vi "Motion@General MotorName Only__Parameter.vi"(1 "ParamterIn":string) -> (0 "ParamterOut":string)   [LabVIEW 2019]
panel:
  in  "Delay":string(combo)
  in  "MotorSelect":string(combo)
  in  "Confirm":bool
  # "Motor@Stop/GetPos/GetState $Motor"
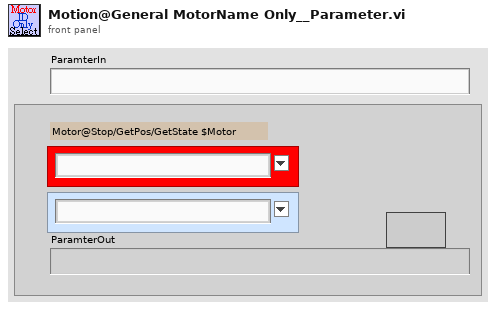
[diagram p1: front panel]
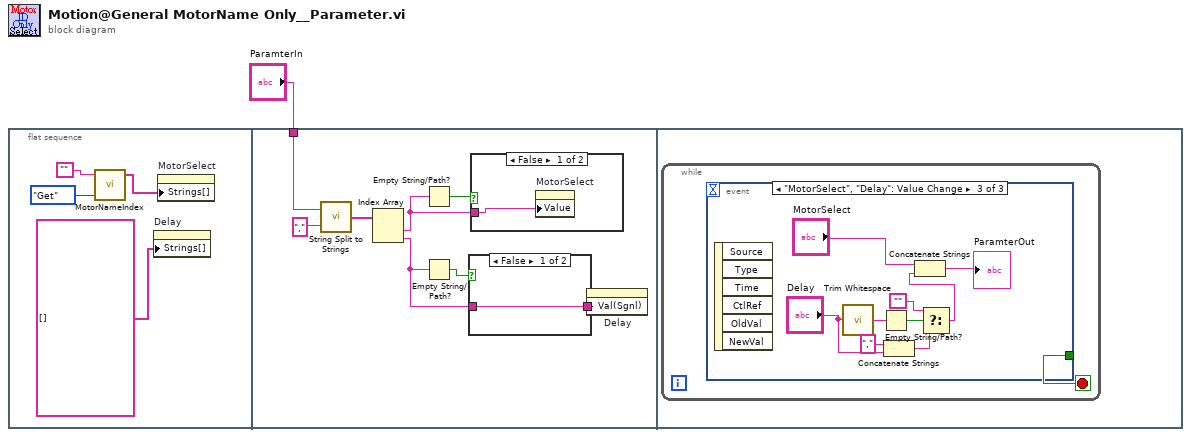
[diagram p0: block diagram]
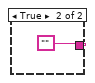
[diagram p2: hidden frame]
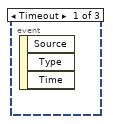
[diagram p4: hidden frame]
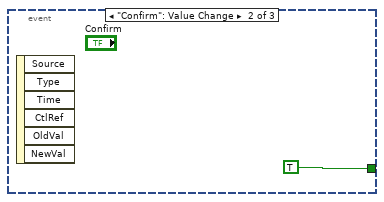
[diagram p5: hidden frame]
diagram:
  n1 = flat-sequence {
    tunnel: "ParamterIn" -> [w11]
    frame #0 {
      n2 = call "MotorNameIndex.vi"("OP"=enum16{"Get", "Update", "Init"}."Get", "MotorName"="") -> ("MotorList"=w2:string[])  [unwired: 1 in, 2 out]
      n3 = property on="Delay" class="CmbBox"("Strings[]"=string[] [] ("Strings []")) -> ()  [unwired: 2 in, 2 out]
      n4 = property on="MotorSelect" class="CmbBox"("Strings[]"=w2) -> ()  [unwired: 2 in, 2 out]
    }
    frame #1 {
      n5 = call "String Split to Strings.vi"("search string/char (-)"=",", "String"=w11) -> ("Array"=w13:string[])
      n6 = Index Array(array=w13) -> (element #1=w9:string, element #2=w6:string)  [unwired: 2 in]
      n7 = Empty String/Path?(string/path=w9) -> (empty?=w10:bool)
      n8 = Empty String/Path?(string/path=w6) -> (empty?=w8:bool)
      n9 = case shown="False" w8 {
        tunnel: [w14 ""] -> w7
        tunnel: w6 -> [w14 _]
        frame False {
        }
        frame True {
        }
      }
      n10 = case shown="False" w10 {
        tunnel: w9 -> [w16 _]
        frame False {
          n11 = property on="MotorSelect" class="CmbBox"("Value"=w16) -> ()  [unwired: 2 in, 2 out]
        }
        frame True {
        }
      }
      n12 = property on="Delay" class="CmbBox"("Val(Sgnl)"=w7) -> ()  [unwired: 2 in, 2 out]
    }
    frame #2 {
      n13 = while {
        stop <- w17 stop-if-true
        n14 = event shown="[2] \"MotorSelect\", \"Delay\": Value Change" {
          selector: _ -> [_ _ _]
          dyn-events: _ -> [_ _ _]
          timeout: _ -> [_ _ _]
          tunnel: [_ TRUE _] -> w17
          event Timeout {
            n15 = event-data() -> ()  [unwired: 1 in, 3 out]
          }
          event "Confirm": Value Change {
            n16 = event-data() -> ()  [unwired: 1 in, 6 out]
          }
          event "MotorSelect", "Delay": Value Change {
            n17 = event-data() -> ()  [unwired: 1 in, 6 out]
            n18 = call <vilib>:"Trim Whitespace.vi"("string"="Delay") -> ("trimmed string"=w21:string)  [unwired: 1 in]
            n19 = Empty String/Path?(string/path=w21) -> (empty?=w22:bool)
            n20 = Concatenate Strings("," ("string"), "Delay") -> (w24:string)
            n21 = Select(t="", s=w22, f=w24) -> (s? t:f=w19:string)
            n22 = Concatenate Strings("MotorSelect", w19) -> (→"ParamterOut":string)
          }
        }
      }
    }
  }
